vi "Read Header Value.vi"(8 "error in (no error)":errorcluster, 10 "Header Name":string, 11 "HTTPHeaders_NET in":refnum<class "HttpHeaders_NET.lvclass">) -> (0 "error out":errorcluster, 1 "Header Value":string[](array[string]), 2 "Header Name Out":string, 3 "HTTPHeaders_NET out":refnum<class "HttpHeaders_NET.lvclass">, 4 "Found":bool)   [LabVIEW 2018, in "HttpClient_NET.lvlib" / "HttpHeaders_NET.lvclass"]
doc: "<b> </b> <b> </b>\nHttpClient_NET\nJustin Young - Viviota\nCopyright (c) 2021\nLicense: BSD"
uses:
  HttpHeaders_NET.lvclass
  HttpHeaders_NET.lvclass/HttpHeaders_NET.ctl
  Accessors/Read NET_HttpHeaders.vi
  System.Net.Http
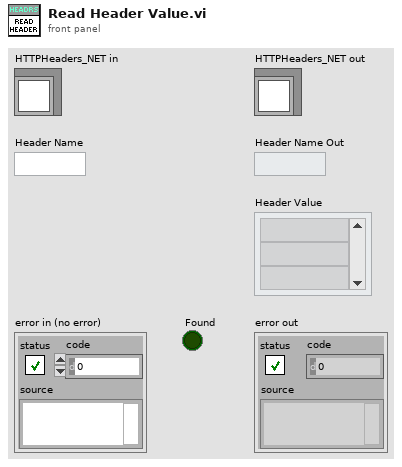
[diagram p1: front panel]
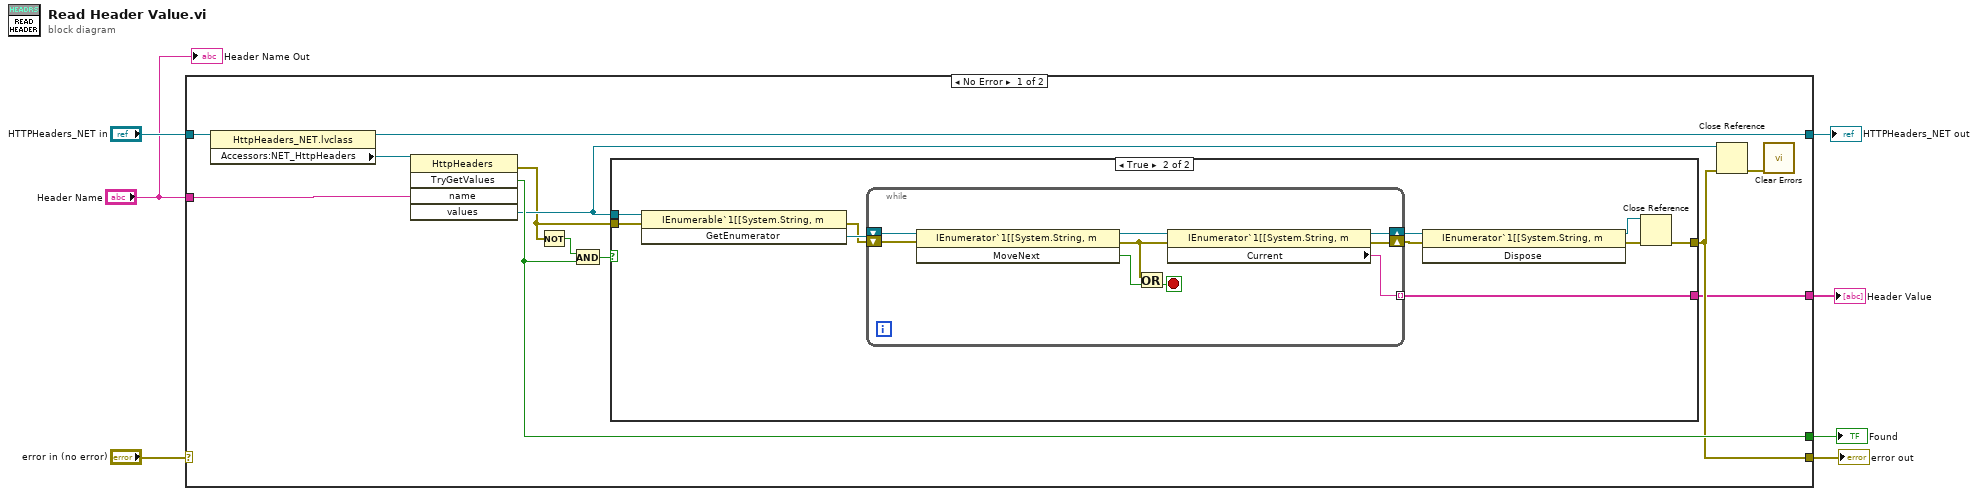
[diagram p0: block diagram]
diagram:
  n1 = case shown="No Error" "error in (no error)" {
    selector: "error in (no error)" -> [_ w41]
    tunnel: [w11 w41] -> w6
    tunnel: [w18 w40] -> w4
    tunnel: "HTTPHeaders_NET in" -> [w19 w40]
    tunnel: [w14 _] -> w3
    tunnel: [w9 _] -> w2
    tunnel: "Header Name" -> [w8 _]
    frame No Error {
      n2 = property class="HttpHeaders_NET.lvclass"(reference=w19) -> (reference out=w18:refnum<class "HttpHeaders_NET.lvclass">, "Accessors:NET_HttpHeaders"=w17:refnum<k24>)  [unwired: 1 in, 1 out]
      n3 = invoke class="HttpHeaders" method="TryGetValues"(reference=w17, "name"=w8) -> (error out=w10:errorcluster, "TryGetValues"=w14:bool, "values"=w13:refnum<k24>)  [unwired: 3 in, 2 out]
      n4 = Not(x=w10) -> (.not. x?=w15:bool)
      n5 = And(x=w15, y=w14) -> (x .and. y?=w16:bool)
      n6 = case shown="True" w16 {
        tunnel: w13 -> [_ w29]
        tunnel: [_ w28] -> w9
        tunnel: [w20 w23] -> w11
        tunnel: w10 -> [w20 w21]
        frame False {
        }
        frame True {
          n7 = invoke class="IEnumerable`1[[System.String, m" method="GetEnumerator"(reference=w29, error in=w21) -> (error out=w22:errorcluster, "GetEnumerator"=w30:refnum<k24>)  [unwired: 1 in, 1 out]
          n8 = while {
            shift-right: [w37] -> w24
            shift-left: w30 -> [w38]
            shift-right: [w33] -> w25
            shift-left: w22 -> [w31]
            tunnel: [w32] -> w28 mode=indexing
            stop <- w35 stop-if-true
            n9 = invoke class="IEnumerator`1[[System.String, m" method="MoveNext"(reference=w38, error in=w31) -> (reference out=w39:refnum<k24>, error out=w34:errorcluster, "MoveNext"=w36:bool)  [unwired: 1 in]
            n10 = Or(x=w34, y=w36) -> (x .or. y?=w35:bool)
            n11 = property class="IEnumerator`1[[System.String, m"(reference=w39, error in=w34) -> (reference out=w37:refnum<k24>, error out=w33:errorcluster, "Current"=w32:string)
          }
          n12 = invoke class="IEnumerator`1[[System.String, m" method="Dispose"(reference=w24, error in=w25) -> (reference out=w26:refnum<k24>, error out=w27:errorcluster)  [unwired: 1 in, 1 out]
          n13 = Close Reference(reference=w26, error in (no error)=w27) -> (error out=w23:errorcluster)
        }
      }
      n14 = Close Reference(reference=w13, error in (no error)=w11) -> (error out=w12:errorcluster)
      n15 = call <vilib>:"Clear Errors.vi"("error in (no error)"=w12) -> ()  [unwired: 5 in, 2 out]
    }
    frame Error {
    }
  }
  "error out" <- w6
  "HTTPHeaders_NET out" <- w4
  "Found" <- w3
  "Header Value" <- w2
  "Header Name Out" <- "Header Name"
